vi "Global stack names.vi"() -> ()   [LabVIEW 2023]
uses:
  ctrl defs/ctrl stack - ARMS.ctl
  ctrl defs/ctrl stack - INTAKE SHOOTER.ctl
panel:
  in  "Tab Control":enum32{"INTAKE & SHOOTER", "CLIMBER"}(tab)
  in  "INTAKE SHOOTER stack":T1={"INTAKE STATE"="/INTAKE/STATE", "RUN INTAKE?"="/INTAKE/RUN?", "RUN REVERSE?"="/INTAKE/REVERSE?", "NOTE LOADED?"="/INTAKE/NOTE?", "SHOOTER STATE"="/SHOOTER/STATE", "SHOOTER FIRE?"="/SHOOTER/FIRE?"}
  in  "RIGHT ARMS":T2={"ARM LOCK"="/DB/INTAKE/", "ARM LIMIT EXTEND"="/DB/INTAKE/", "ARM LIMIT RETRACT "="/DB/INTAKE/", "ARM EXTEND "="/DB/INTAKE/", "ARM RETRACT"="/DB/INTAKE/"}
  in  "LEFT ARMS":T2={"ARM LOCK"="/ARMS/LEFT/LOCK", "ARM LIMIT EXTEND"="/ARMS/LEFT/EXTEND", "ARM LIMIT RETRACT "="/ARMS/LEFT/RETRACT", "ARM EXTEND "="/ARMS/LEFT/EXTEND LIMIT", "ARM RETRACT"="/ARMS/LEFT/RETRACT LIMIT"}
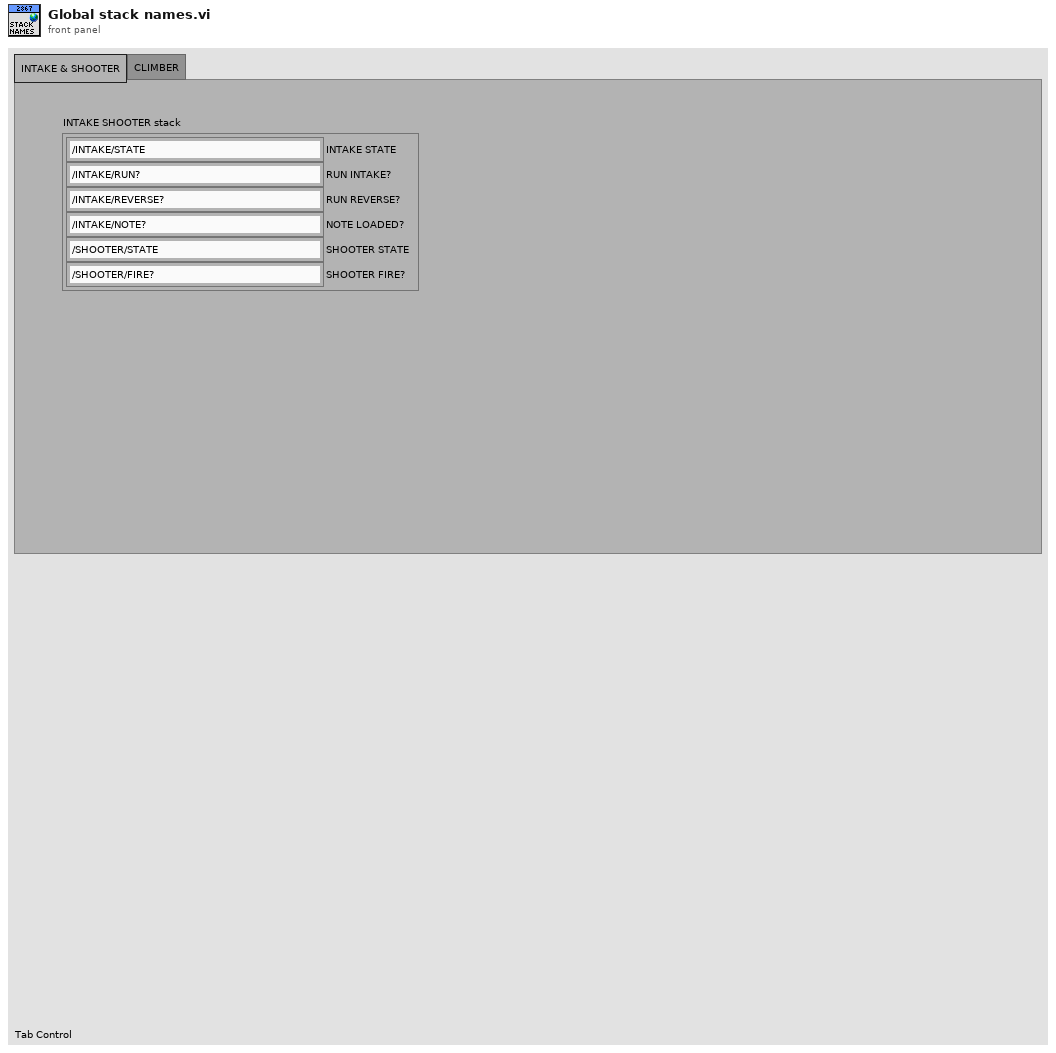
[diagram p1: front panel]
types:
  T1 = typedef "ctrl stack - INTAKE SHOOTER.ctl" = cluster{"INTAKE STATE":string, "RUN INTAKE?":string, "RUN REVERSE?":string, "NOTE LOADED?":string, "SHOOTER STATE":string, "SHOOTER FIRE?":string}
  T2 = typedef "ctrl stack - ARMS.ctl" = cluster{"ARM LOCK":string, "ARM LIMIT EXTEND":string, "ARM LIMIT RETRACT ":string, "ARM EXTEND ":string, "ARM RETRACT":string}
diagram:
